vi "ke37xx Blender Trigger Control.vi"(0 "VISA Resource Name":refnum<visa-resource-name>, 5 "Action (0: Clear)":enum16{"Clear", "Wait"}(ring), 7 "Blender (1)":u8=1 min=1 max=2, 9 "Timeout Seconds (2 sec)":dbl=2.0, 11 "error in (no error)":errorcluster) -> (4 "VISA Resource Name Out":refnum<visa-resource-name>, 8 "Triggered":bool, 15 "error out":errorcluster)   [LabVIEW 2009, in "Keithley 3700 Series.lvlib"]
doc: "This VI allows you to clear the blender event detector or wait on the blender to enter the detected state."
uses:
  <instrlib>/Keithley 3706/Keithley 3700 Series.lvlib
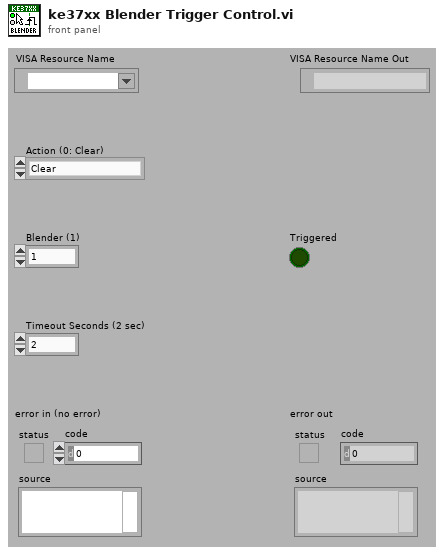
[diagram p1: front panel]
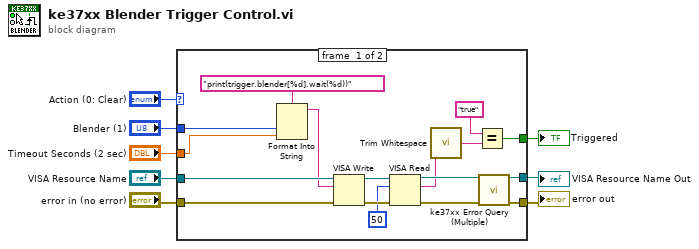
[diagram p0: block diagram]
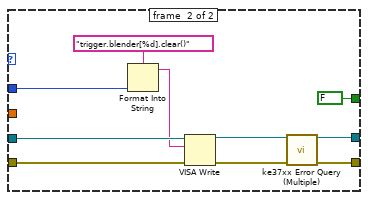
[diagram p2: hidden frame]
diagram:
  n1 = case shown="\"Clear\"" "Action (0: Clear)" {
    tunnel: [w25 w35] -> w8
    tunnel: [w24 w34] -> w7
    tunnel: "VISA Resource Name" -> [w23 w33]
    tunnel: "error in (no error)" -> [w22 w32]
    tunnel: "Blender (1)" -> [w15 w30]
    tunnel: "Timeout Seconds (2 sec)" -> [w14 _]
    tunnel: [w9 FALSE] -> w1
    frame #0 {
      n2 = Format Into String(format string="print(trigger.blender[%d].wait(%d))", w15, w14) -> (resulting string=w13:string)  [unwired: 2 in, 1 out]
      n3 = VISA Write(VISA resource name=w23, write buffer=w13, error in (no error)=w22) -> (VISA resource name out=w20:refnum<visa-resource-name>, error out=w21:errorcluster)  [unwired: 1 out]
      n4 = VISA Read(VISA resource name=w20, byte count=u32 50, error in (no error)=w21) -> (VISA resource name out=w19:refnum<visa-resource-name>, read buffer=w12:string, error out=w18:errorcluster)  [unwired: 1 out]
      n5 = call <vilib>:"Trim Whitespace.vi"("string"=w12) -> ("trimmed string"=w11:string)  [unwired: 1 in]
      n6 = Equal?(x="true", y=w11) -> (x = y?=w9:bool)
      n7 = call <instrlib>:"ke37xx Error Query (Multiple).vi"("VISA resource name"=w19, "error in (no error)"=w18) -> ("VISA resource name out"=w25:refnum<visa-resource-name>, "error out"=w24:errorcluster)  [unwired: 12 out]
    }
    frame #1 {
      n8 = Format Into String(format string="trigger.blender[%d].clear()", w30) -> (resulting string=w29:string)  [unwired: 2 in, 1 out]
      n9 = VISA Write(VISA resource name=w33, write buffer=w29, error in (no error)=w32) -> (VISA resource name out=w28:refnum<visa-resource-name>, error out=w27:errorcluster)  [unwired: 1 out]
      n10 = call <instrlib>:"ke37xx Error Query (Multiple).vi"("VISA resource name"=w28, "error in (no error)"=w27) -> ("VISA resource name out"=w35:refnum<visa-resource-name>, "error out"=w34:errorcluster)  [unwired: 12 out]
    }
  }
  "VISA Resource Name Out" <- w8
  "error out" <- w7
  "Triggered" <- w1
